vi "相机2初始化.vi"() -> (1 "Session Out":T2, 2 "Image":T1, 3 "相机状态":bool, 4 "error out":errorcluster)   [LabVIEW 2014]
uses:
  <vilib>/userdefined/High Color/IMAQdx.ctl
  <vilib>/vision/Image Controls.llb/IMAQ Image.ctl
  Controls/MsgAction.ctl
  <vilib>/vision/driver/IMAQdx.llb/IMAQdx Camera Control Mode.ctl
  Global.vi
  <vilib>/vision/driver/NI_Vision_Acquisition_Software.lvlib
panel:
  out "error out 2":errorcluster
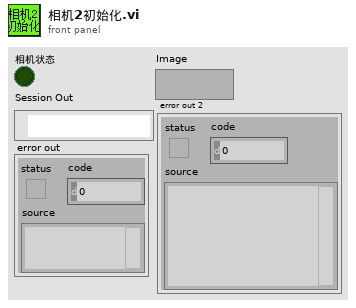
[diagram p1: front panel]
types:
  T1 = typedef "IMAQ Image.ctl" = refnum<image>
  T2 = typedef "IMAQdx.ctl" = refnum<k21>
  T3 = typedef "NI_Vision_Acquisition_Software.lvlib/IMAQdx Camera Control Mode.ctl" = enum32{"Controller", "Listener"}
  T4 = typedef "MsgAction.ctl" = enum16{"初始化", "添加消息", "区分结果添加消息", "清空消息", "获取消息"}
  T5 = typedef "OtherSpec.ctl" = cluster{"其它勾选类规格":T6, "其它数据类规格":T7, "相机名称":T8}
  T6 = typedef "其它勾选类规格.ctl" = cluster{"保存NG图片":bool, "保存OK图片":bool, "保存数据":bool, "开机默认开启监控摄像头":bool}
  T7 = typedef "其他数据类规格.ctl" = cluster{"相机1像素-毫米换算系数":dbl, "相机2像素-毫米换算系数":dbl, "D盘剩余空间预警(G)":dbl, "视频最长录制时间(秒)":dbl}
  T8 = typedef "相机名称品牌使用状态.ctl" = cluster{"相机1名称":T2, "相机2名称":T2, "Cam1启用":bool, "Cam2启用":bool, "Basler1":bool, "Basler2":bool}
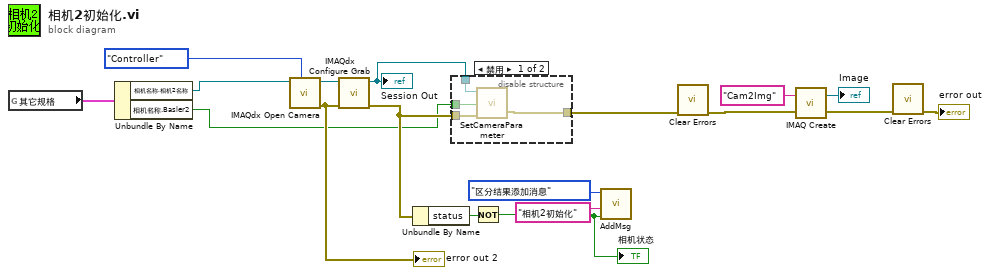
[diagram p0: block diagram]
diagram:
  n1 = global read "Global.vi" "其它规格"() -> (w12:T5)
  n2 = Unbundle By Name(w12) -> ("相机名称.相机2名称"=w2:T2, "相机名称.Basler2"=w3:bool)
  n3 = call <vilib>:"IMAQdx Open Camera.vi"("Camera Control Mode"=IMAQdx_Camera_Control_Mode."Controller", "Session In"=w2) -> ("error out"=w17:errorcluster, "Session Out"=w16:T2)  [unwired: 8 in]
  "error out 2" <- w17
  n4 = call <vilib>:"IMAQdx Configure Grab.vi"("error in"=w17, "Session In"=w16) -> ("error out"=w6:errorcluster, "Session Out"=w5:T2)  [unwired: 8 in]
  "Session Out" <- w5
  n5 = Unbundle By Name(w6) -> ("status"=w13:bool)
  n6 = disable-structure shown="禁用" {
    disable-tunnel: w6 -> [w22 w23]
    disable-tunnel: w5 -> [w21 _]
    disable-tunnel: [w20 w23] -> w4
    disable-tunnel: w3 -> [w19 _]
    frame Disabled {
      n7 = call "SetCameraParameter.vi"("error in"=w22, "相机品牌为Basler?"=w19, "Session In"=w21) -> ("error out"=w20:errorcluster)  [unwired: 1 in, 1 out]
    }
    frame Enabled {
    }
  }
  n8 = Not(x=w13) -> (.not. x?=w18:bool)
  "相机状态" <- w18
  n9 = call "AddMsg.vi"("Result"=w18, "添加消息"="相机2初始化" ("消息显示"), "消息Action"=MsgAction."区分结果添加消息") -> ()  [unwired: 1 in, 1 out]
  n10 = call <vilib>:"Clear Errors.vi"("error in (no error)"=w4) -> ("error out"=w7:errorcluster)  [unwired: 5 in, 1 out]
  n11 = call "IMAQ Create"("Image Name"="Cam2Img", "error in (no error)"=w7) -> ("New Image"=→"Image":T1, "error out"=w10:errorcluster)  [unwired: 3 in]
  n12 = call <vilib>:"Clear Errors.vi"("error in (no error)"=w10) -> ("error out"=→"error out":errorcluster)  [unwired: 5 in, 1 out]
